vi "Generate_Random_Params.vi"(8 "Amplitude Range":cluster{"max":dbl, "min":dbl}={"max"=50.0, "min"=150.0}, 10 "Duration Range":cluster{"max":dbl, "min":dbl}={"max"=600.0, "min"=200.0}, 11 "Samples":i32=3000) -> (0 "Duration":i32[](array[numeric]), 1 "Amplitude":dbl[](array[numeric]), 2 "Position":dbl[](array[numeric]))   [LabVIEW 2020]
uses:
  <vilib>/Analysis/1siggen.llb/Ramp Pattern by Samples.vi
  <vilib>/Analysis/NI_AALBase.lvlib
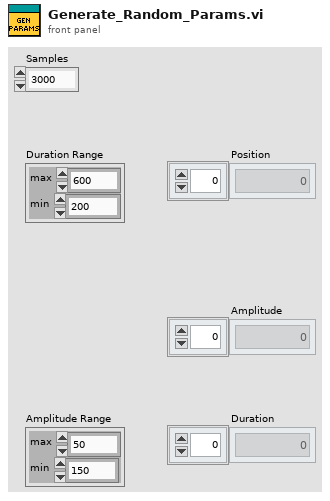
[diagram p1: front panel]
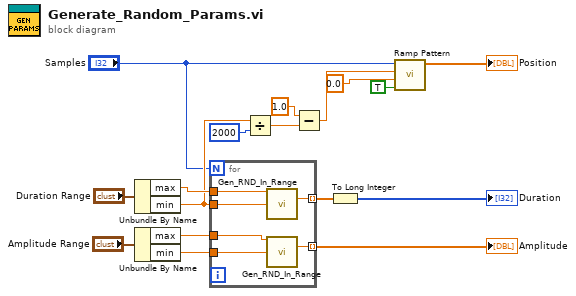
[diagram p0: block diagram]
diagram:
  n1 = Unbundle By Name("Duration Range") -> ("max"=w17:dbl, "min"=w16:dbl)
  n2 = Unbundle By Name("Amplitude Range") -> ("max"=w13:dbl, "min"=w14:dbl)
  n3 = for {
    N: "Samples" -> [_]
    tunnel: w14 -> [w23]
    tunnel: w13 -> [w22]
    tunnel: w17 -> [w21]
    tunnel: w16 -> [w20]
    tunnel: [w19] -> w9 mode=indexing
    tunnel: [w18] -> w10 mode=indexing
    n4 = call "Gen_RND_In_Range.vi"("Upper Bound"=w21, "Lower Bound"=w20) -> ("RND_In_Range"=w18:dbl)  [unwired: 13 in]
    n5 = call "Gen_RND_In_Range.vi"("Upper Bound"=w22, "Lower Bound"=w23) -> ("RND_In_Range"=w19:dbl)  [unwired: 13 in]
  }
  "Amplitude" <- w9
  n6 = Divide(x=w16, y=2000 ("samples")) -> (x/y=w5:dbl)
  n7 = Subtract(x=1.0 ("end"), y=w5) -> (x-y=w6:dbl)
  n8 = To Long Integer(number=w10) -> (32bit integer=→"Duration":i32[])
  n9 = call-poly <vilib>:"Ramp Pattern.vi"("exclude end?"=TRUE, "start"=0.0 ("end"), "end"=w6, "samples"="Samples") -> ("Ramp Pattern"=→"Position":dbl[])  [unwired: 6 in, 1 out]
